vi "check_whether_configuration_exists.vi"(8 "error in (no error)":errorcluster, 10 "configuration name":string, 11 "GenericPlugin in":refnum<class "GenericComponent.lvclass">) -> (0 "error out":errorcluster, 2 "exists?":bool, 3 "GenericPlugin out":refnum<class "GenericComponent.lvclass">)   [LabVIEW 2010, in "GenericComponent.lvclass"]
uses:
  GenericComponent.lvclass
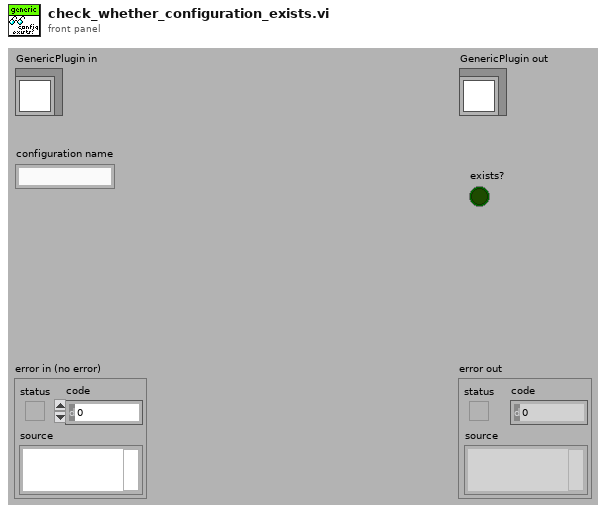
[diagram p1: front panel]
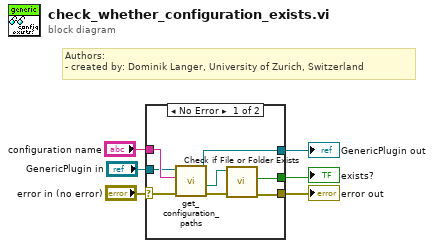
[diagram p0: block diagram]
diagram:
  # "Authors: \n- created by: Dominik Langer, University of Zurich, Switzerland"
  n1 = case shown="No Error" "error in (no error)" {
    selector: "error in (no error)" -> [w11 w16]
    tunnel: [w14 w16] -> w5
    tunnel: [w8 w15] -> w3
    tunnel: "GenericPlugin in" -> [w10 w15]
    tunnel: "configuration name" -> [w12 _]
    tunnel: [w13 _] -> w1
    frame No Error {
      n2 = call-dynamic "get_configuration_paths.vi"("error in (no error)"=w11, "file name (without ending)"=w12, "GenericComponent in"=w10) -> ("error out"=w9:errorcluster, "configuration file path"=w7:path, "GenericComponent out"=w8:refnum<class "GenericComponent.lvclass">)  [unwired: 1 in, 5 out]
      n3 = call <vilib>:"Check if File or Folder Exists.vi"("error in (no error)"=w9, "path"=w7) -> ("error out"=w14:errorcluster, "file or folder exists?"=w13:bool)  [unwired: 7 in, 1 out]
    }
    frame Error {
    }
  }
  "error out" <- w5
  "GenericPlugin out" <- w3
  "exists?" <- w1
